vi "Write password.vi"(8 "error in (no error)":errorcluster, 10 "password":string, 11 "SetEngineerAccessMode in":refnum<class "SetEngineerAccessMode.lvclass">) -> (0 "error out":errorcluster, 3 "SetEngineerAccessMode out":refnum<class "SetEngineerAccessMode.lvclass">)   [LabVIEW 2022 SP3, in "TCSDataDefinitions.lvlib" / "TCSCommand.lvlib" / "SetAccessMode.lvlib" / "SetEngineerAccessMode.lvclass"]
uses:
  SetEngineerAccessMode.lvclass
  SetEngineerAccessMode.lvclass/SetEngineerAccessMode.ctl
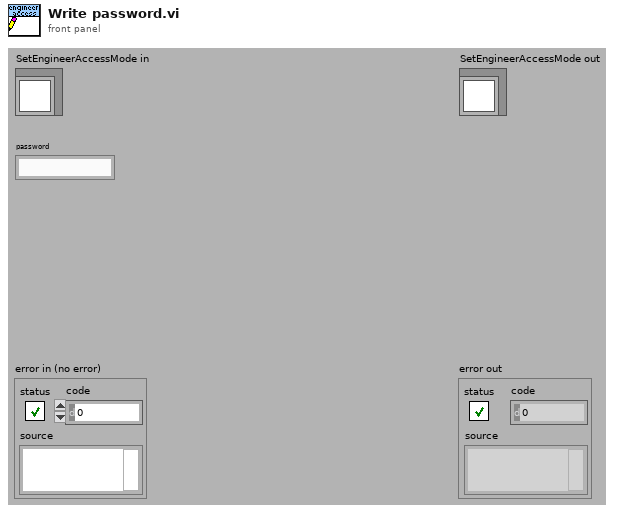
[diagram p1: front panel]
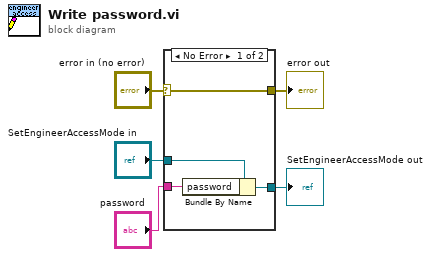
[diagram p0: block diagram]
diagram:
  n1 = case shown="No Error" "error in (no error)" {
    selector: "error in (no error)" -> [w9 w10]
    tunnel: [w9 w10] -> w4
    tunnel: [w7 w11] -> w2
    tunnel: "SetEngineerAccessMode in" -> [w8 w11]
    tunnel: "password" -> [w6 _]
    frame No Error {
      n2 = Bundle By Name(cluster=w8, "password"=w6) -> (w7:refnum<class "SetEngineerAccessMode.lvclass">)
    }
    frame Error {
    }
  }
  "error out" <- w4
  "SetEngineerAccessMode out" <- w2
